vi "Project XML Editor.vi"() -> ()   [LabVIEW 2019]
uses:
  Project XML Editor/TypeDefs/Dependency Parameters.ctl
  Project XML Editor/Project XML Editor.lvclass
panel:
  out "Array":T1[](array[typedef])
  out "error out":errorcluster
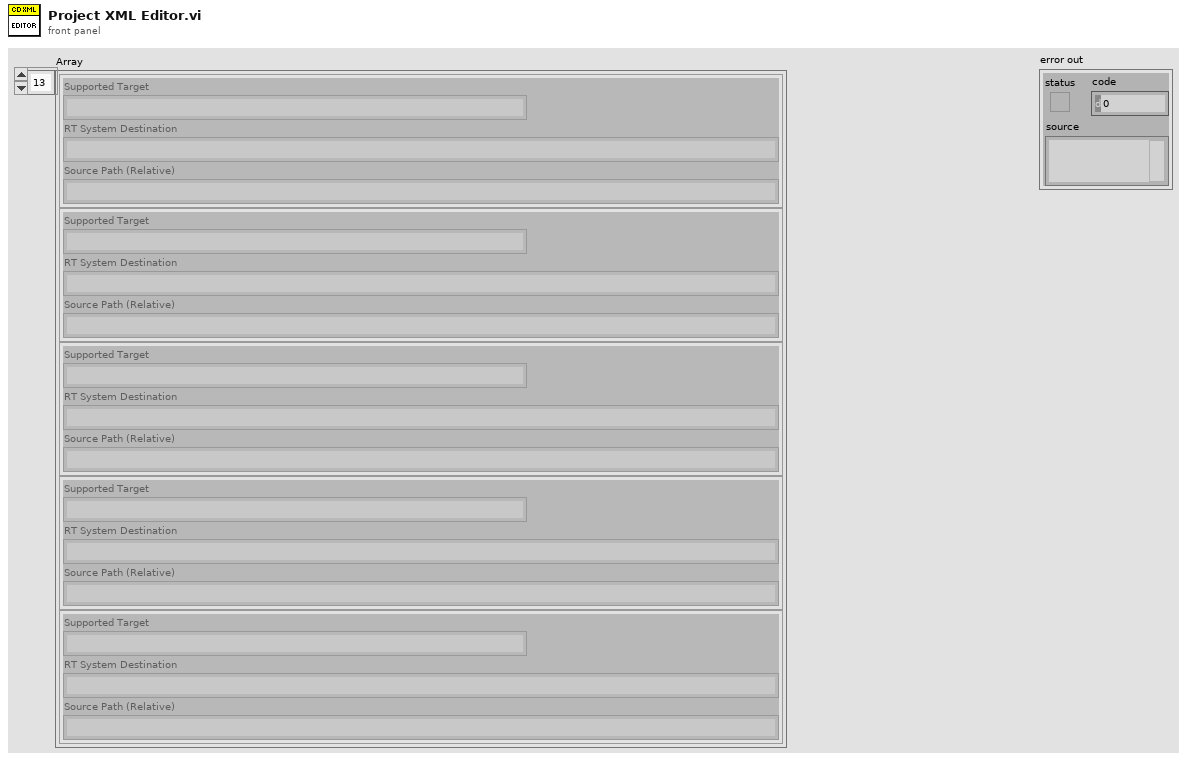
[diagram p1: front panel]
types:
  T1 = typedef "Project XML Editor.lvclass/Dependency Parameters.ctl" = cluster{"Supported Target":string, "RT System Destination":string, "Source Path (Relative)":string}
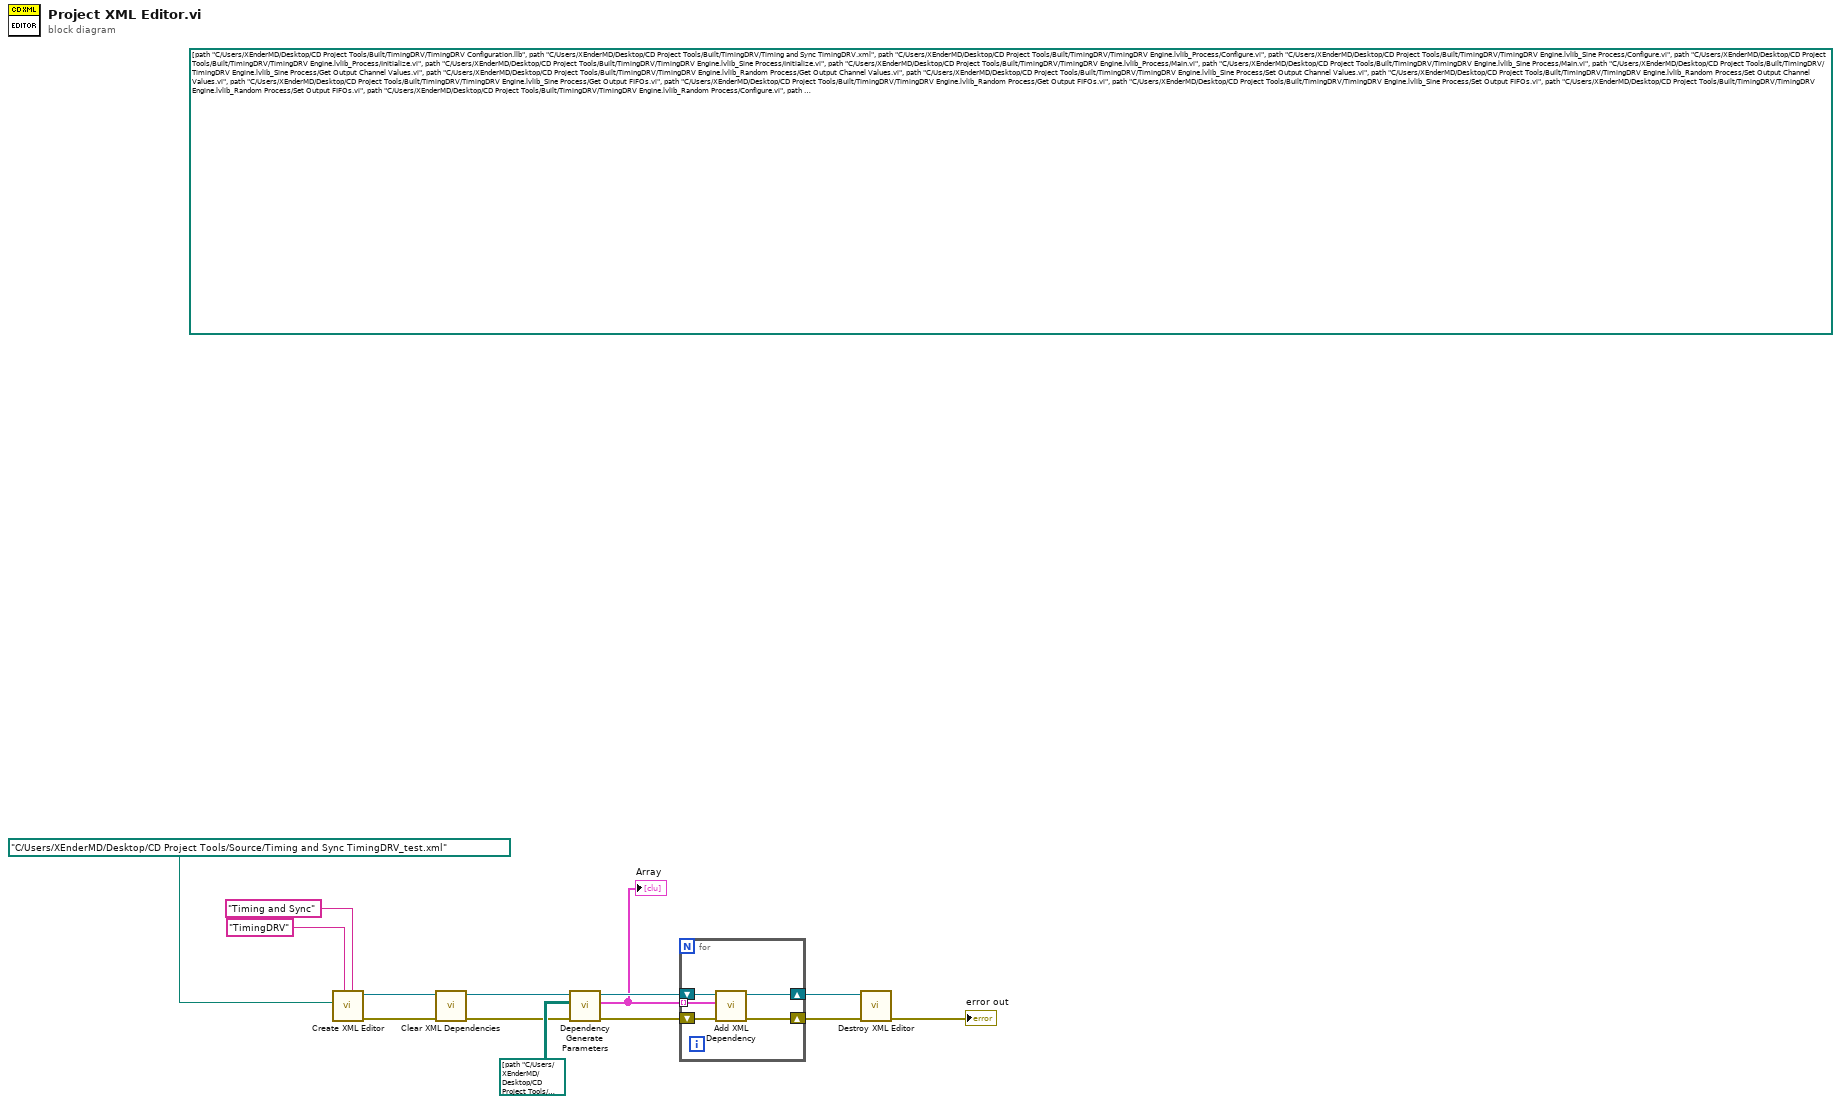
[diagram p0: block diagram]
diagram:
  (unwired) path[][] [[path "C:/Users/XEnderMD/Desktop/CD Project Tools/Built/TimingDRV/TimingDRV Configuration.llb", path "C:/Users/XEnderMD/Desktop/CD Project Tools/Built/TimingDRV/Timing and Sync TimingDRV.xml", path "C:/Users/XEnderMD/Desktop/CD Project Tools/Built/TimingDRV/TimingDRV Engine.lvlib_Process/Configure.vi", path "C:/Users/XEnderMD/Desktop/CD Project Tools/Built/TimingDRV/TimingDRV Engine.lvlib_Sine Process/Configure.vi", path "C:/Users/XEnderMD/Desktop/CD Project Tools/Built/TimingDRV/TimingDRV Engine.lvlib_Process/Initialize.vi", path "C:/Users/XEnderMD/Desktop/CD Project Tools/Built/TimingDRV/TimingDRV Engine.lvlib_Sine Process/Initialize.vi", path "C:/Users/XEnderMD/Desktop/CD Project Tools/Built/TimingDRV/TimingDRV Engine.lvlib_Process/Main.vi", path "C:/Users/XEnderMD/Desktop/CD Project Tools/Built/TimingDRV/TimingDRV Engine.lvlib_Sine Process/Main.vi", path "C:/Users/XEnderMD/Desktop/CD Project Tools/Built/TimingDRV/TimingDRV Engine.lvlib_Sine Process/Get Output Channel Values.vi", path "C:/Users/XEnderMD/Desktop/CD Project Tools/Built/TimingDRV/TimingDRV Engine.lvlib_Random Process/Get Output Channel Values.vi", path "C:/Users/XEnderMD/Desktop/CD Project Tools/Built/TimingDRV/TimingDRV Engine.lvlib_Sine Process/Set Output Channel Values.vi", path "C:/Users/XEnderMD/Desktop/CD Project Tools/Built/TimingDRV/TimingDRV Engine.lvlib_Random Process/Set Output Channel Values.vi", path "C:/Users/XEnderMD/Desktop/CD Project Tools/Built/TimingDRV/TimingDRV Engine.lvlib_Sine Process/Get Output FIFOs.vi", path "C:/Users/XEnderMD/Desktop/CD Project Tools/Built/TimingDRV/TimingDRV Engine.lvlib_Random Process/Get Output FIFOs.vi", path "C:/Users/XEnderMD/Desktop/CD Project Tools/Built/TimingDRV/TimingDRV Engine.lvlib_Sine Process/Set Output FIFOs.vi", path "C:/Users/XEnderMD/Desktop/CD Project Tools/Built/TimingDRV/TimingDRV Engine.lvlib_Random Process/Set Output FIFOs.vi", path "C:/Users/XEnderMD/Desktop/CD Project Tools/Built/TimingDRV/TimingDRV Engine.lvlib_Random Process/Configure.vi", path "C:/Users/XEnderMD/Desktop/CD Project Tools/Built/TimingDRV/TimingDRV Engine.lvlib_Random Process/Initialize.vi", path "C:/Users/XEnderMD/Desktop/CD Project Tools/Built/TimingDRV/TimingDRV Engine.lvlib_Sine Process/Initialize Output Channel Values.vi", path "C:/Users/XEnderMD/Desktop/CD Project Tools/Built/TimingDRV/TimingDRV Engine.lvlib_Random Process/Initialize Output Channel Values.vi", path "C:/Users/XEnderMD/Desktop/CD Project Tools/Built/TimingDRV/TimingDRV Engine.lvlib_Random Process/Main.vi", path "C:/Users/XEnderMD/Desktop/CD Project Tools/Built/TimingDRV/TimingDRV Engine.lvlib_Sine Process/Update Channel Value.vi", path "C:/Users/XEnderMD/Desktop/CD Project Tools/Built/TimingDRV/TimingDRV Engine.lvlib_Random Process/Update Channel Value.vi", path "", path "", path "", path "", path "", path "", path "", path "", path "", path "", path "", path "", path "", path "", path "", path "", path ""], [path "C:/Users/XEnderMD/Desktop/CD Project Tools/Built/TimingDRV/Windows/TimingDRV Engine Windows.llb", path "C:/Users/XEnderMD/Desktop/CD Project Tools/Built/TimingDRV/Windows/TimingDRV Engine.lvlib_Assembler/Main.vi", path "C:/Users/XEnderMD/Desktop/CD Project Tools/Built/TimingDRV/Windows/TimingDRV Engine.lvlib_Input Process/Main.vi", path "C:/Users/XEnderMD/Desktop/CD Project Tools/Built/TimingDRV/Windows/TimingDRV Engine.lvlib_Output Process/Initialize Output Channel Values.vi", path "C:/Users/XEnderMD/Desktop/CD Project Tools/Built/TimingDRV/Windows/TimingDRV Engine.lvlib_Sine Process/Initialize Output Channel Values.vi", path "C:/Users/XEnderMD/Desktop/CD Project Tools/Built/TimingDRV/Windows/TimingDRV Engine.lvlib_Output Process/Update Channel Value.vi", path "C:/Users/XEnderMD/Desktop/CD Project Tools/Built/TimingDRV/Windows/TimingDRV Engine.lvlib_Sine Process/Update Channel Value.vi", path "C:/Users/XEnderMD/Desktop/CD Project Tools/Built/TimingDRV/Windows/TimingDRV Engine.lvlib_Random Process/Initialize Output Channel Values.vi", path "C:/Users/XEnderMD/Desktop/CD Project Tools/Built/TimingDRV/Windows/TimingDRV Engine.lvlib_Random Process/Update Channel Value.vi", path "C:/Users/XEnderMD/Desktop/CD Project Tools/Built/TimingDRV/Windows/TimingDRV Engine.lvlib_Assembler/Configure.vi", path "C:/Users/XEnderMD/Desktop/CD Project Tools/Built/TimingDRV/Windows/TimingDRV Engine.lvlib_Output Process/Configure.vi", path "C:/Users/XEnderMD/Desktop/CD Project Tools/Built/TimingDRV/Windows/TimingDRV Engine.lvlib_Assembler/Initialize.vi", path "C:/Users/XEnderMD/Desktop/CD Project Tools/Built/TimingDRV/Windows/TimingDRV Engine.lvlib_Output Process/Initialize.vi", path "C:/Users/XEnderMD/Desktop/CD Project Tools/Built/TimingDRV/Windows/TimingDRV Engine.lvlib_Output Process/Main.vi", path "C:/Users/XEnderMD/Desktop/CD Project Tools/Built/TimingDRV/Windows/TimingDRV Engine.lvlib_Output Process/Get Output Channel Values.vi", path "C:/Users/XEnderMD/Desktop/CD Project Tools/Built/TimingDRV/Windows/TimingDRV Engine.lvlib_Sine Process/Get Output Channel Values.vi", path "C:/Users/XEnderMD/Desktop/CD Project Tools/Built/TimingDRV/Windows/TimingDRV Engine.lvlib_Output Process/Set Output Channel Values.vi", path "C:/Users/XEnderMD/Desktop/CD Project Tools/Built/TimingDRV/Windows/TimingDRV Engine.lvlib_Sine Process/Set Output Channel Values.vi", path "C:/Users/XEnderMD/Desktop/CD Project Tools/Built/TimingDRV/Windows/TimingDRV Engine.lvlib_Output Process/Get Output FIFOs.vi", path "C:/Users/XEnderMD/Desktop/CD Project Tools/Built/TimingDRV/Windows/TimingDRV Engine.lvlib_Sine Process/Get Output FIFOs.vi", path "C:/Users/XEnderMD/Desktop/CD Project Tools/Built/TimingDRV/Windows/TimingDRV Engine.lvlib_Output Process/Set Output FIFOs.vi", path "C:/Users/XEnderMD/Desktop/CD Project Tools/Built/TimingDRV/Windows/TimingDRV Engine.lvlib_Sine Process/Set Output FIFOs.vi", path "C:/Users/XEnderMD/Desktop/CD Project Tools/Built/TimingDRV/Windows/TimingDRV Engine.lvlib_Sine Process/Configure.vi", path "C:/Users/XEnderMD/Desktop/CD Project Tools/Built/TimingDRV/Windows/TimingDRV Engine.lvlib_Sine Process/Initialize.vi", path "C:/Users/XEnderMD/Desktop/CD Project Tools/Built/TimingDRV/Windows/TimingDRV Engine.lvlib_Sine Process/Main.vi", path "C:/Users/XEnderMD/Desktop/CD Project Tools/Built/TimingDRV/Windows/TimingDRV Engine.lvlib_Random Process/Get Output Channel Values.vi", path "C:/Users/XEnderMD/Desktop/CD Project Tools/Built/TimingDRV/Windows/TimingDRV Engine.lvlib_Random Process/Set Output Channel Values.vi", path "C:/Users/XEnderMD/Desktop/CD Project Tools/Built/TimingDRV/Windows/TimingDRV Engine.lvlib_Random Process/Get Output FIFOs.vi", path "C:/Users/XEnderMD/Desktop/CD Project Tools/Built/TimingDRV/Windows/TimingDRV Engine.lvlib_Random Process/Set Output FIFOs.vi", path "C:/Users/XEnderMD/Desktop/CD Project Tools/Built/TimingDRV/Windows/TimingDRV Engine.lvlib_Random Process/Configure.vi", path "C:/Users/XEnderMD/Desktop/CD Project Tools/Built/TimingDRV/Windows/TimingDRV Engine.lvlib_Random Process/Initialize.vi", path "C:/Users/XEnderMD/Desktop/CD Project Tools/Built/TimingDRV/Windows/TimingDRV Engine.lvlib_Random Process/Main.vi", path "C:/Users/XEnderMD/Desktop/CD Project Tools/Built/TimingDRV/Windows/TimingDRV Engine.lvlib_Process/Configure.vi", path "C:/Users/XEnderMD/Desktop/CD Project Tools/Built/TimingDRV/Windows/TimingDRV Engine.lvlib_Assembler/Launcher.vi", path "C:/Users/XEnderMD/Desktop/CD Project Tools/Built/TimingDRV/Windows/TimingDRV Engine.lvlib_Process/Launcher.vi", path "C:/Users/XEnderMD/Desktop/CD Project Tools/Built/TimingDRV/Windows/TimingDRV Engine.lvlib_Process/Initialize.vi", path "C:/Users/XEnderMD/Desktop/CD Project Tools/Built/TimingDRV/Windows/TimingDRV Engine.lvlib_Process/Main.vi", path "C:/Users/XEnderMD/Desktop/CD Project Tools/Built/TimingDRV/Windows/TimingDRV Engine.lvlib_Assembler/Shutdown.vi", path "C:/Users/XEnderMD/Desktop/CD Project Tools/Built/TimingDRV/Windows/TimingDRV Engine.lvlib_Process/Shutdown.vi", path ""], [path "C:/Users/XEnderMD/Desktop/CD Project Tools/Built/TimingDRV/Pharlap/TimingDRV Engine Pharlap.llb", path "C:/Users/XEnderMD/Desktop/CD Project Tools/Built/TimingDRV/Pharlap/TimingDRV Engine.lvlib_Assembler/Main.vi", path "C:/Users/XEnderMD/Desktop/CD Project Tools/Built/TimingDRV/Pharlap/TimingDRV Engine.lvlib_Input Process/Main.vi", path "C:/Users/XEnderMD/Desktop/CD Project Tools/Built/TimingDRV/Pharlap/TimingDRV Engine.lvlib_Output Process/Initialize Output Channel Values.vi", path "C:/Users/XEnderMD/Desktop/CD Project Tools/Built/TimingDRV/Pharlap/TimingDRV Engine.lvlib_Sine Process/Initialize Output Channel Values.vi", path "C:/Users/XEnderMD/Desktop/CD Project Tools/Built/TimingDRV/Pharlap/TimingDRV Engine.lvlib_Output Process/Update Channel Value.vi", path "C:/Users/XEnderMD/Desktop/CD Project Tools/Built/TimingDRV/Pharlap/TimingDRV Engine.lvlib_Sine Process/Update Channel Value.vi", path "C:/Users/XEnderMD/Desktop/CD Project Tools/Built/TimingDRV/Pharlap/TimingDRV Engine.lvlib_Random Process/Initialize Output Channel Values.vi", path "C:/Users/XEnderMD/Desktop/CD Project Tools/Built/TimingDRV/Pharlap/TimingDRV Engine.lvlib_Random Process/Update Channel Value.vi", path "C:/Users/XEnderMD/Desktop/CD Project Tools/Built/TimingDRV/Pharlap/TimingDRV Engine.lvlib_Assembler/Configure.vi", path "C:/Users/XEnderMD/Desktop/CD Project Tools/Built/TimingDRV/Pharlap/TimingDRV Engine.lvlib_Output Process/Configure.vi", path "C:/Users/XEnderMD/Desktop/CD Project Tools/Built/TimingDRV/Pharlap/TimingDRV Engine.lvlib_Assembler/Initialize.vi", path "C:/Users/XEnderMD/Desktop/CD Project Tools/Built/TimingDRV/Pharlap/TimingDRV Engine.lvlib_Output Process/Initialize.vi", path "C:/Users/XEnderMD/Desktop/CD Project Tools/Built/TimingDRV/Pharlap/TimingDRV Engine.lvlib_Output Process/Main.vi", path "C:/Users/XEnderMD/Desktop/CD Project Tools/Built/TimingDRV/Pharlap/TimingDRV Engine.lvlib_Output Process/Get Output Channel Values.vi", path "C:/Users/XEnderMD/Desktop/CD Project Tools/Built/TimingDRV/Pharlap/TimingDRV Engine.lvlib_Sine Process/Get Output Channel Values.vi", path "C:/Users/XEnderMD/Desktop/CD Project Tools/Built/TimingDRV/Pharlap/TimingDRV Engine.lvlib_Output Process/Set Output Channel Values.vi", path "C:/Users/XEnderMD/Desktop/CD Project Tools/Built/TimingDRV/Pharlap/TimingDRV Engine.lvlib_Sine Process/Set Output Channel Values.vi", path "C:/Users/XEnderMD/Desktop/CD Project Tools/Built/TimingDRV/Pharlap/TimingDRV Engine.lvlib_Output Process/Get Output FIFOs.vi", path "C:/Users/XEnderMD/Desktop/CD Project Tools/Built/TimingDRV/Pharlap/TimingDRV Engine.lvlib_Sine Process/Get Output FIFOs.vi", path "C:/Users/XEnderMD/Desktop/CD Project Tools/Built/TimingDRV/Pharlap/TimingDRV Engine.lvlib_Output Process/Set Output FIFOs.vi", path "C:/Users/XEnderMD/Desktop/CD Project Tools/Built/TimingDRV/Pharlap/TimingDRV Engine.lvlib_Sine Process/Set Output FIFOs.vi", path "C:/Users/XEnderMD/Desktop/CD Project Tools/Built/TimingDRV/Pharlap/TimingDRV Engine.lvlib_Sine Process/Configure.vi", path "C:/Users/XEnderMD/Desktop/CD Project Tools/Built/TimingDRV/Pharlap/TimingDRV Engine.lvlib_Sine Process/Initialize.vi", path "C:/Users/XEnderMD/Desktop/CD Project Tools/Built/TimingDRV/Pharlap/TimingDRV Engine.lvlib_Sine Process/Main.vi", path "C:/Users/XEnderMD/Desktop/CD Project Tools/Built/TimingDRV/Pharlap/TimingDRV Engine.lvlib_Random Process/Get Output Channel Values.vi", path "C:/Users/XEnderMD/Desktop/CD Project Tools/Built/TimingDRV/Pharlap/TimingDRV Engine.lvlib_Random Process/Set Output Channel Values.vi", path "C:/Users/XEnderMD/Desktop/CD Project Tools/Built/TimingDRV/Pharlap/TimingDRV Engine.lvlib_Random Process/Get Output FIFOs.vi", path "C:/Users/XEnderMD/Desktop/CD Project Tools/Built/TimingDRV/Pharlap/TimingDRV Engine.lvlib_Random Process/Set Output FIFOs.vi", path "C:/Users/XEnderMD/Desktop/CD Project Tools/Built/TimingDRV/Pharlap/TimingDRV Engine.lvlib_Random Process/Configure.vi", path "C:/Users/XEnderMD/Desktop/CD Project Tools/Built/TimingDRV/Pharlap/TimingDRV Engine.lvlib_Random Process/Initialize.vi", path "C:/Users/XEnderMD/Desktop/CD Project Tools/Built/TimingDRV/Pharlap/TimingDRV Engine.lvlib_Random Process/Main.vi", path "C:/Users/XEnderMD/Desktop/CD Project Tools/Built/TimingDRV/Pharlap/TimingDRV Engine.lvlib_Process/Configure.vi", path "C:/Users/XEnderMD/Desktop/CD Project Tools/Built/TimingDRV/Pharlap/TimingDRV Engine.lvlib_Assembler/Launcher.vi", path "C:/Users/XEnderMD/Desktop/CD Project Tools/Built/TimingDRV/Pharlap/TimingDRV Engine.lvlib_Process/Launcher.vi", path "C:/Users/XEnderMD/Desktop/CD Project Tools/Built/TimingDRV/Pharlap/TimingDRV Engine.lvlib_Process/Initialize.vi", path "C:/Users/XEnderMD/Desktop/CD Project Tools/Built/TimingDRV/Pharlap/TimingDRV Engine.lvlib_Process/Main.vi", path "C:/Users/XEnderMD/Desktop/CD Project Tools/Built/TimingDRV/Pharlap/TimingDRV Engine.lvlib_Assembler/Shutdown.vi", path "C:/Users/XEnderMD/Desktop/CD Project Tools/Built/TimingDRV/Pharlap/TimingDRV Engine.lvlib_Process/Shutdown.vi", path "C:/Users/XEnderMD/Desktop/CD Project Tools/Built/TimingDRV/Engine Release_depinstr.bin"], [path "C:/Users/XEnderMD/Desktop/CD Project Tools/Built/TimingDRV/VxWorks/TimingDRV Engine VxWorks.llb", path "C:/Users/XEnderMD/Desktop/CD Project Tools/Built/TimingDRV/VxWorks/TimingDRV Engine.lvlib_Assembler/Main.vi", path "C:/Users/XEnderMD/Desktop/CD Project Tools/Built/TimingDRV/VxWorks/TimingDRV Engine.lvlib_Input Process/Main.vi", path "C:/Users/XEnderMD/Desktop/CD Project Tools/Built/TimingDRV/VxWorks/TimingDRV Engine.lvlib_Output Process/Initialize Output Channel Values.vi", path "C:/Users/XEnderMD/Desktop/CD Project Tools/Built/TimingDRV/VxWorks/TimingDRV Engine.lvlib_Sine Process/Initialize Output Channel Values.vi", path "C:/Users/XEnderMD/Desktop/CD Project Tools/Built/TimingDRV/VxWorks/TimingDRV Engine.lvlib_Output Process/Update Channel Value.vi", path "C:/Users/XEnderMD/Desktop/CD Project Tools/Built/TimingDRV/VxWorks/TimingDRV Engine.lvlib_Sine Process/Update Channel Value.vi", path "C:/Users/XEnderMD/Desktop/CD Project Tools/Built/TimingDRV/VxWorks/TimingDRV Engine.lvlib_Random Process/Initialize Output Channel Values.vi", path "C:/Users/XEnderMD/Desktop/CD Project Tools/Built/TimingDRV/VxWorks/TimingDRV Engine.lvlib_Random Process/Update Channel Value.vi", path "C:/Users/XEnderMD/Desktop/CD Project Tools/Built/TimingDRV/VxWorks/TimingDRV Engine.lvlib_Assembler/Configure.vi", path "C:/Users/XEnderMD/Desktop/CD Project Tools/Built/TimingDRV/VxWorks/TimingDRV Engine.lvlib_Output Process/Configure.vi", path "C:/Users/XEnderMD/Desktop/CD Project Tools/Built/TimingDRV/VxWorks/TimingDRV Engine.lvlib_Assembler/Initialize.vi", path "C:/Users/XEnderMD/Desktop/CD Project Tools/Built/TimingDRV/VxWorks/TimingDRV Engine.lvlib_Output Process/Initialize.vi", path "C:/Users/XEnderMD/Desktop/CD Project Tools/Built/TimingDRV/VxWorks/TimingDRV Engine.lvlib_Output Process/Main.vi", path "C:/Users/XEnderMD/Desktop/CD Project Tools/Built/TimingDRV/VxWorks/TimingDRV Engine.lvlib_Output Process/Get Output Channel Values.vi", path "C:/Users/XEnderMD/Desktop/CD Project Tools/Built/TimingDRV/VxWorks/TimingDRV Engine.lvlib_Sine Process/Get Output Channel Values.vi", path "C:/Users/XEnderMD/Desktop/CD Project Tools/Built/TimingDRV/VxWorks/TimingDRV Engine.lvlib_Output Process/Set Output Channel Values.vi", path "C:/Users/XEnderMD/Desktop/CD Project Tools/Built/TimingDRV/VxWorks/TimingDRV Engine.lvlib_Sine Process/Set Output Channel Values.vi", path "C:/Users/XEnderMD/Desktop/CD Project Tools/Built/TimingDRV/VxWorks/TimingDRV Engine.lvlib_Output Process/Get Output FIFOs.vi", path "C:/Users/XEnderMD/Desktop/CD Project Tools/Built/TimingDRV/VxWorks/TimingDRV Engine.lvlib_Sine Process/Get Output FIFOs.vi", path "C:/Users/XEnderMD/Desktop/CD Project Tools/Built/TimingDRV/VxWorks/TimingDRV Engine.lvlib_Output Process/Set Output FIFOs.vi", path "C:/Users/XEnderMD/Desktop/CD Project Tools/Built/TimingDRV/VxWorks/TimingDRV Engine.lvlib_Sine Process/Set Output FIFOs.vi", path "C:/Users/XEnderMD/Desktop/CD Project Tools/Built/TimingDRV/VxWorks/TimingDRV Engine.lvlib_Sine Process/Configure.vi", path "C:/Users/XEnderMD/Desktop/CD Project Tools/Built/TimingDRV/VxWorks/TimingDRV Engine.lvlib_Sine Process/Initialize.vi", path "C:/Users/XEnderMD/Desktop/CD Project Tools/Built/TimingDRV/VxWorks/TimingDRV Engine.lvlib_Sine Process/Main.vi", path "C:/Users/XEnderMD/Desktop/CD Project Tools/Built/TimingDRV/VxWorks/TimingDRV Engine.lvlib_Random Process/Get Output Channel Values.vi", path "C:/Users/XEnderMD/Desktop/CD Project Tools/Built/TimingDRV/VxWorks/TimingDRV Engine.lvlib_Random Process/Set Output Channel Values.vi", path "C:/Users/XEnderMD/Desktop/CD Project Tools/Built/TimingDRV/VxWorks/TimingDRV Engine.lvlib_Random Process/Get Output FIFOs.vi", path "C:/Users/XEnderMD/Desktop/CD Project Tools/Built/TimingDRV/VxWorks/TimingDRV Engine.lvlib_Random Process/Set Output FIFOs.vi", path "C:/Users/XEnderMD/Desktop/CD Project Tools/Built/TimingDRV/VxWorks/TimingDRV Engine.lvlib_Random Process/Configure.vi", path "C:/Users/XEnderMD/Desktop/CD Project Tools/Built/TimingDRV/VxWorks/TimingDRV Engine.lvlib_Random Process/Initialize.vi", path "C:/Users/XEnderMD/Desktop/CD Project Tools/Built/TimingDRV/VxWorks/TimingDRV Engine.lvlib_Random Process/Main.vi", path "C:/Users/XEnderMD/Desktop/CD Project Tools/Built/TimingDRV/VxWorks/TimingDRV Engine.lvlib_Process/Configure.vi", path "C:/Users/XEnderMD/Desktop/CD Project Tools/Built/TimingDRV/VxWorks/TimingDRV Engine.lvlib_Assembler/Launcher.vi", path "C:/Users/XEnderMD/Desktop/CD Project Tools/Built/TimingDRV/VxWorks/TimingDRV Engine.lvlib_Process/Launcher.vi", path "C:/Users/XEnderMD/Desktop/CD Project Tools/Built/TimingDRV/VxWorks/TimingDRV Engine.lvlib_Process/Initialize.vi", path "C:/Users/XEnderMD/Desktop/CD Project Tools/Built/TimingDRV/VxWorks/TimingDRV Engine.lvlib_Process/Main.vi", path "C:/Users/XEnderMD/Desktop/CD Project Tools/Built/TimingDRV/VxWorks/TimingDRV Engine.lvlib_Assembler/Shutdown.vi", path "C:/Users/XEnderMD/Desktop/CD Project Tools/Built/TimingDRV/VxWorks/TimingDRV Engine.lvlib_Process/Shutdown.vi", path "C:/Users/XEnderMD/Desktop/CD Project Tools/Built/TimingDRV/Engine Release_depinstr.bin"], [path "C:/Users/XEnderMD/Desktop/CD Project Tools/Built/TimingDRV/Linux_32_ARM/TimingDRV Engine LinuxARM.llb", path "C:/Users/XEnderMD/Desktop/CD Project Tools/Built/TimingDRV/Linux_32_ARM/TimingDRV Engine.lvlib_Assembler/Main.vi", path "C:/Users/XEnderMD/Desktop/CD Project Tools/Built/TimingDRV/Linux_32_ARM/TimingDRV Engine.lvlib_Input Process/Main.vi", path "C:/Users/XEnderMD/Desktop/CD Project Tools/Built/TimingDRV/Linux_32_ARM/TimingDRV Engine.lvlib_Output Process/Initialize Output Channel Values.vi", path "C:/Users/XEnderMD/Desktop/CD Project Tools/Built/TimingDRV/Linux_32_ARM/TimingDRV Engine.lvlib_Sine Process/Initialize Output Channel Values.vi", path "C:/Users/XEnderMD/Desktop/CD Project Tools/Built/TimingDRV/Linux_32_ARM/TimingDRV Engine.lvlib_Output Process/Update Channel Value.vi", path "C:/Users/XEnderMD/Desktop/CD Project Tools/Built/TimingDRV/Linux_32_ARM/TimingDRV Engine.lvlib_Sine Process/Update Channel Value.vi", path "C:/Users/XEnderMD/Desktop/CD Project Tools/Built/TimingDRV/Linux_32_ARM/TimingDRV Engine.lvlib_Random Process/Initialize Output Channel Values.vi", path "C:/Users/XEnderMD/Desktop/CD Project Tools/Built/TimingDRV/Linux_32_ARM/TimingDRV Engine.lvlib_Random Process/Update Channel Value.vi", path "C:/Users/XEnderMD/Desktop/CD Project Tools/Built/TimingDRV/Linux_32_ARM/TimingDRV Engine.lvlib_Assembler/Configure.vi", path "C:/Users/XEnderMD/Desktop/CD Project Tools/Built/TimingDRV/Linux_32_ARM/TimingDRV Engine.lvlib_Output Process/Configure.vi", path "C:/Users/XEnderMD/Desktop/CD Project Tools/Built/TimingDRV/Linux_32_ARM/TimingDRV Engine.lvlib_Assembler/Initialize.vi", path "C:/Users/XEnderMD/Desktop/CD Project Tools/Built/TimingDRV/Linux_32_ARM/TimingDRV Engine.lvlib_Output Process/Initialize.vi", path "C:/Users/XEnderMD/Desktop/CD Project Tools/Built/TimingDRV/Linux_32_ARM/TimingDRV Engine.lvlib_Output Process/Main.vi", path "C:/Users/XEnderMD/Desktop/CD Project Tools/Built/TimingDRV/Linux_32_ARM/TimingDRV Engine.lvlib_Output Process/Get Output Channel Values.vi", path "C:/Users/XEnderMD/Desktop/CD Project Tools/Built/TimingDRV/Linux_32_ARM/TimingDRV Engine.lvlib_Sine Process/Get Output Channel Values.vi", path "C:/Users/XEnderMD/Desktop/CD Project Tools/Built/TimingDRV/Linux_32_ARM/TimingDRV Engine.lvlib_Output Process/Set Output Channel Values.vi", path "C:/Users/XEnderMD/Desktop/CD Project Tools/Built/TimingDRV/Linux_32_ARM/TimingDRV Engine.lvlib_Sine Process/Set Output Channel Values.vi", path "C:/Users/XEnderMD/Desktop/CD Project Tools/Built/TimingDRV/Linux_32_ARM/TimingDRV Engine.lvlib_Output Process/Get Output FIFOs.vi", path "C:/Users/XEnderMD/Desktop/CD Project Tools/Built/TimingDRV/Linux_32_ARM/TimingDRV Engine.lvlib_Sine Process/Get Output FIFOs.vi", path "C:/Users/XEnderMD/Desktop/CD Project Tools/Built/TimingDRV/Linux_32_ARM/TimingDRV Engine.lvlib_Output Process/Set Output FIFOs.vi", path "C:/Users/XEnderMD/Desktop/CD Project Tools/Built/TimingDRV/Linux_32_ARM/TimingDRV Engine.lvlib_Sine Process/Set Output FIFOs.vi", path "C:/Users/XEnderMD/Desktop/CD Project Tools/Built/TimingDRV/Linux_32_ARM/TimingDRV Engine.lvlib_Sine Process/Configure.vi", path "C:/Users/XEnderMD/Desktop/CD Project Tools/Built/TimingDRV/Linux_32_ARM/TimingDRV Engine.lvlib_Sine Process/Initialize.vi", path "C:/Users/XEnderMD/Desktop/CD Project Tools/Built/TimingDRV/Linux_32_ARM/TimingDRV Engine.lvlib_Sine Process/Main.vi", path "C:/Users/XEnderMD/Desktop/CD Project Tools/Built/TimingDRV/Linux_32_ARM/TimingDRV Engine.lvlib_Random Process/Get Output Channel Values.vi", path "C:/Users/XEnderMD/Desktop/CD Project Tools/Built/TimingDRV/Linux_32_ARM/TimingDRV Engine.lvlib_Random Process/Set Output Channel Values.vi", path "C:/Users/XEnderMD/Desktop/CD Project Tools/Built/TimingDRV/Linux_32_ARM/TimingDRV Engine.lvlib_Random Process/Get Output FIFOs.vi", path "C:/Users/XEnderMD/Desktop/CD Project Tools/Built/TimingDRV/Linux_32_ARM/TimingDRV Engine.lvlib_Random Process/Set Output FIFOs.vi", path "C:/Users/XEnderMD/Desktop/CD Project Tools/Built/TimingDRV/Linux_32_ARM/TimingDRV Engine.lvlib_Random Process/Configure.vi", path "C:/Users/XEnderMD/Desktop/CD Project Tools/Built/TimingDRV/Linux_32_ARM/TimingDRV Engine.lvlib_Random Process/Initialize.vi", path "C:/Users/XEnderMD/Desktop/CD Project Tools/Built/TimingDRV/Linux_32_ARM/TimingDRV Engine.lvlib_Random Process/Main.vi", path "C:/Users/XEnderMD/Desktop/CD Project Tools/Built/TimingDRV/Linux_32_ARM/TimingDRV Engine.lvlib_Process/Configure.vi", path "C:/Users/XEnderMD/Desktop/CD Project Tools/Built/TimingDRV/Linux_32_ARM/TimingDRV Engine.lvlib_Assembler/Launcher.vi", path "C:/Users/XEnderMD/Desktop/CD Project Tools/Built/TimingDRV/Linux_32_ARM/TimingDRV Engine.lvlib_Process/Launcher.vi", path "C:/Users/XEnderMD/Desktop/CD Project Tools/Built/TimingDRV/Linux_32_ARM/TimingDRV Engine.lvlib_Process/Initialize.vi", path "C:/Users/XEnderMD/Desktop/CD Project Tools/Built/TimingDRV/Linux_32_ARM/TimingDRV Engine.lvlib_Process/Main.vi", path "C:/Users/XEnderMD/Desktop/CD Project Tools/Built/TimingDRV/Linux_32_ARM/TimingDRV Engine.lvlib_Assembler/Shutdown.vi", path "C:/Users/XEnderMD/Desktop/CD Project Tools/Built/TimingDRV/Linux_32_ARM/TimingDRV Engine.lvlib_Process/Shutdown.vi", path "C:/Users/XEnderMD/Desktop/CD Project Tools/Built/TimingDRV/Engine Release_depinstr.bin"], [path "C:/Users/XEnderMD/Desktop/CD Project Tools/Built/TimingDRV/Linux_x64/TimingDRV Engine Linux64.llb", path "C:/Users/XEnderMD/Desktop/CD Project Tools/Built/TimingDRV/Linux_x64/TimingDRV Engine.lvlib_Assembler/Main.vi", path "C:/Users/XEnderMD/Desktop/CD Project Tools/Built/TimingDRV/Linux_x64/TimingDRV Engine.lvlib_Input Process/Main.vi", path "C:/Users/XEnderMD/Desktop/CD Project Tools/Built/TimingDRV/Linux_x64/TimingDRV Engine.lvlib_Output Process/Initialize Output Channel Values.vi", path "C:/Users/XEnderMD/Desktop/CD Project Tools/Built/TimingDRV/Linux_x64/TimingDRV Engine.lvlib_Sine Process/Initialize Output Channel Values.vi", path "C:/Users/XEnderMD/Desktop/CD Project Tools/Built/TimingDRV/Linux_x64/TimingDRV Engine.lvlib_Output Process/Update Channel Value.vi", path "C:/Users/XEnderMD/Desktop/CD Project Tools/Built/TimingDRV/Linux_x64/TimingDRV Engine.lvlib_Sine Process/Update Channel Value.vi", path "C:/Users/XEnderMD/Desktop/CD Project Tools/Built/TimingDRV/Linux_x64/TimingDRV Engine.lvlib_Random Process/Initialize Output Channel Values.vi", path "C:/Users/XEnderMD/Desktop/CD Project Tools/Built/TimingDRV/Linux_x64/TimingDRV Engine.lvlib_Random Process/Update Channel Value.vi", path "C:/Users/XEnderMD/Desktop/CD Project Tools/Built/TimingDRV/Linux_x64/TimingDRV Engine.lvlib_Assembler/Configure.vi", path "C:/Users/XEnderMD/Desktop/CD Project Tools/Built/TimingDRV/Linux_x64/TimingDRV Engine.lvlib_Output Process/Configure.vi", path "C:/Users/XEnderMD/Desktop/CD Project Tools/Built/TimingDRV/Linux_x64/TimingDRV Engine.lvlib_Assembler/Initialize.vi", path "C:/Users/XEnderMD/Desktop/CD Project Tools/Built/TimingDRV/Linux_x64/TimingDRV Engine.lvlib_Output Process/Initialize.vi", path "C:/Users/XEnderMD/Desktop/CD Project Tools/Built/TimingDRV/Linux_x64/TimingDRV Engine.lvlib_Output Process/Main.vi", path "C:/Users/XEnderMD/Desktop/CD Project Tools/Built/TimingDRV/Linux_x64/TimingDRV Engine.lvlib_Output Process/Get Output Channel Values.vi", path "C:/Users/XEnderMD/Desktop/CD Project Tools/Built/TimingDRV/Linux_x64/TimingDRV Engine.lvlib_Sine Process/Get Output Channel Values.vi", path "C:/Users/XEnderMD/Desktop/CD Project Tools/Built/TimingDRV/Linux_x64/TimingDRV Engine.lvlib_Output Process/Set Output Channel Values.vi", path "C:/Users/XEnderMD/Desktop/CD Project Tools/Built/TimingDRV/Linux_x64/TimingDRV Engine.lvlib_Sine Process/Set Output Channel Values.vi", path "C:/Users/XEnderMD/Desktop/CD Project Tools/Built/TimingDRV/Linux_x64/TimingDRV Engine.lvlib_Output Process/Get Output FIFOs.vi", path "C:/Users/XEnderMD/Desktop/CD Project Tools/Built/TimingDRV/Linux_x64/TimingDRV Engine.lvlib_Sine Process/Get Output FIFOs.vi", path "C:/Users/XEnderMD/Desktop/CD Project Tools/Built/TimingDRV/Linux_x64/TimingDRV Engine.lvlib_Output Process/Set Output FIFOs.vi", path "C:/Users/XEnderMD/Desktop/CD Project Tools/Built/TimingDRV/Linux_x64/TimingDRV Engine.lvlib_Sine Process/Set Output FIFOs.vi", path "C:/Users/XEnderMD/Desktop/CD Project Tools/Built/TimingDRV/Linux_x64/TimingDRV Engine.lvlib_Sine Process/Configure.vi", path "C:/Users/XEnderMD/Desktop/CD Project Tools/Built/TimingDRV/Linux_x64/TimingDRV Engine.lvlib_Sine Process/Initialize.vi", path "C:/Users/XEnderMD/Desktop/CD Project Tools/Built/TimingDRV/Linux_x64/TimingDRV Engine.lvlib_Sine Process/Main.vi", path "C:/Users/XEnderMD/Desktop/CD Project Tools/Built/TimingDRV/Linux_x64/TimingDRV Engine.lvlib_Random Process/Get Output Channel Values.vi", path "C:/Users/XEnderMD/Desktop/CD Project Tools/Built/TimingDRV/Linux_x64/TimingDRV Engine.lvlib_Random Process/Set Output Channel Values.vi", path "C:/Users/XEnderMD/Desktop/CD Project Tools/Built/TimingDRV/Linux_x64/TimingDRV Engine.lvlib_Random Process/Get Output FIFOs.vi", path "C:/Users/XEnderMD/Desktop/CD Project Tools/Built/TimingDRV/Linux_x64/TimingDRV Engine.lvlib_Random Process/Set Output FIFOs.vi", path "C:/Users/XEnderMD/Desktop/CD Project Tools/Built/TimingDRV/Linux_x64/TimingDRV Engine.lvlib_Random Process/Configure.vi", path "C:/Users/XEnderMD/Desktop/CD Project Tools/Built/TimingDRV/Linux_x64/TimingDRV Engine.lvlib_Random Process/Initialize.vi", path "C:/Users/XEnderMD/Desktop/CD Project Tools/Built/TimingDRV/Linux_x64/TimingDRV Engine.lvlib_Random Process/Main.vi", path "C:/Users/XEnderMD/Desktop/CD Project Tools/Built/TimingDRV/Linux_x64/TimingDRV Engine.lvlib_Process/Configure.vi", path "C:/Users/XEnderMD/Desktop/CD Project Tools/Built/TimingDRV/Linux_x64/TimingDRV Engine.lvlib_Assembler/Launcher.vi", path "C:/Users/XEnderMD/Desktop/CD Project Tools/Built/TimingDRV/Linux_x64/TimingDRV Engine.lvlib_Process/Launcher.vi", path "C:/Users/XEnderMD/Desktop/CD Project Tools/Built/TimingDRV/Linux_x64/TimingDRV Engine.lvlib_Process/Initialize.vi", path "C:/Users/XEnderMD/Desktop/CD Project Tools/Built/TimingDRV/Linux_x64/TimingDRV Engine.lvlib_Process/Main.vi", path "C:/Users/XEnderMD/Desktop/CD Project Tools/Built/TimingDRV/Linux_x64/TimingDRV Engine.lvlib_Assembler/Shutdown.vi", path "C:/Users/XEnderMD/Desktop/CD Project Tools/Built/TimingDRV/Linux_x64/TimingDRV Engine.lvlib_Process/Shutdown.vi", path "C:/Users/XEnderMD/Desktop/CD Project Tools/Built/TimingDRV/Engine Release_depinstr.bin"]] ("Generated files 2")
  n1 = call "Create XML Editor.vi"("Common Doc Dir"="Timing and Sync", "CD Name"="TimingDRV", "XML Path"=path "C:/Users/XEnderMD/Desktop/CD Project Tools/Source/Timing and Sync TimingDRV_test.xml") -> ("error out"=w8:errorcluster, "Project XML Editor out"=w9:refnum<class "Project XML Editor.lvclass">)  [unwired: 7 in]
  n2 = call "Clear XML Dependencies.vi"("error in (no error)"=w8, "Project XML Editor in"=w9) -> ("error out"=w5:errorcluster, "Project XML Editor out"=w4:refnum<class "Project XML Editor.lvclass">)  [unwired: 8 in]
  n3 = call "Dependency Generate Parameters.vi"("error in (no error)"=w5, "Generated files in"=path[][] [[path "C:/Users/XEnderMD/Desktop/CD Project Tools/Built/TimingDRV/TimingDRV Configuration.llb", path "C:/Users/XEnderMD/Desktop/CD Project Tools/Built/TimingDRV/Timing and Sync TimingDRV.xml", path "C:/Users/XEnderMD/Desktop/CD Project Tools/Built/TimingDRV/TimingDRV Engine.lvlib_Process/Configure.vi", path "C:/Users/XEnderMD/Desktop/CD Project Tools/Built/TimingDRV/TimingDRV Engine.lvlib_Sine Process/Configure.vi", path "C:/Users/XEnderMD/Desktop/CD Project Tools/Built/TimingDRV/TimingDRV Engine.lvlib_Process/Initialize.vi", path "C:/Users/XEnderMD/Desktop/CD Project Tools/Built/TimingDRV/TimingDRV Engine.lvlib_Sine Process/Initialize.vi", path "C:/Users/XEnderMD/Desktop/CD Project Tools/Built/TimingDRV/TimingDRV Engine.lvlib_Process/Main.vi", path "C:/Users/XEnderMD/Desktop/CD Project Tools/Built/TimingDRV/TimingDRV Engine.lvlib_Sine Process/Main.vi", path "C:/Users/XEnderMD/Desktop/CD Project Tools/Built/TimingDRV/TimingDRV Engine.lvlib_Sine Process/Get Output Channel Values.vi", path "C:/Users/XEnderMD/Desktop/CD Project Tools/Built/TimingDRV/TimingDRV Engine.lvlib_Random Process/Get Output Channel Values.vi", path "C:/Users/XEnderMD/Desktop/CD Project Tools/Built/TimingDRV/TimingDRV Engine.lvlib_Sine Process/Set Output Channel Values.vi", path "C:/Users/XEnderMD/Desktop/CD Project Tools/Built/TimingDRV/TimingDRV Engine.lvlib_Random Process/Set Output Channel Values.vi", path "C:/Users/XEnderMD/Desktop/CD Project Tools/Built/TimingDRV/TimingDRV Engine.lvlib_Sine Process/Get Output FIFOs.vi", path "C:/Users/XEnderMD/Desktop/CD Project Tools/Built/TimingDRV/TimingDRV Engine.lvlib_Random Process/Get Output FIFOs.vi", path "C:/Users/XEnderMD/Desktop/CD Project Tools/Built/TimingDRV/TimingDRV Engine.lvlib_Sine Process/Set Output FIFOs.vi", path "C:/Users/XEnderMD/Desktop/CD Project Tools/Built/TimingDRV/TimingDRV Engine.lvlib_Random Process/Set Output FIFOs.vi", path "C:/Users/XEnderMD/Desktop/CD Project Tools/Built/TimingDRV/TimingDRV Engine.lvlib_Random Process/Configure.vi", path "C:/Users/XEnderMD/Desktop/CD Project Tools/Built/TimingDRV/TimingDRV Engine.lvlib_Random Process/Initialize.vi", path "C:/Users/XEnderMD/Desktop/CD Project Tools/Built/TimingDRV/TimingDRV Engine.lvlib_Sine Process/Initialize Output Channel Values.vi", path "C:/Users/XEnderMD/Desktop/CD Project Tools/Built/TimingDRV/TimingDRV Engine.lvlib_Random Process/Initialize Output Channel Values.vi", path "C:/Users/XEnderMD/Desktop/CD Project Tools/Built/TimingDRV/TimingDRV Engine.lvlib_Random Process/Main.vi", path "C:/Users/XEnderMD/Desktop/CD Project Tools/Built/TimingDRV/TimingDRV Engine.lvlib_Sine Process/Update Channel Value.vi", path "C:/Users/XEnderMD/Desktop/CD Project Tools/Built/TimingDRV/TimingDRV Engine.lvlib_Random Process/Update Channel Value.vi", path "", path "", path "", path "", path "", path "", path "", path "", path "", path "", path "", path "", path "", path "", path "", path "", path ""], [path "C:/Users/XEnderMD/Desktop/CD Project Tools/Built/TimingDRV/Windows/TimingDRV Engine Windows.llb", path "C:/Users/XEnderMD/Desktop/CD Project Tools/Built/TimingDRV/Windows/TimingDRV Engine.lvlib_Assembler/Main.vi", path "C:/Users/XEnderMD/Desktop/CD Project Tools/Built/TimingDRV/Windows/TimingDRV Engine.lvlib_Input Process/Main.vi", path "C:/Users/XEnderMD/Desktop/CD Project Tools/Built/TimingDRV/Windows/TimingDRV Engine.lvlib_Output Process/Initialize Output Channel Values.vi", path "C:/Users/XEnderMD/Desktop/CD Project Tools/Built/TimingDRV/Windows/TimingDRV Engine.lvlib_Sine Process/Initialize Output Channel Values.vi", path "C:/Users/XEnderMD/Desktop/CD Project Tools/Built/TimingDRV/Windows/TimingDRV Engine.lvlib_Output Process/Update Channel Value.vi", path "C:/Users/XEnderMD/Desktop/CD Project Tools/Built/TimingDRV/Windows/TimingDRV Engine.lvlib_Sine Process/Update Channel Value.vi", path "C:/Users/XEnderMD/Desktop/CD Project Tools/Built/TimingDRV/Windows/TimingDRV Engine.lvlib_Random Process/Initialize Output Channel Values.vi", path "C:/Users/XEnderMD/Desktop/CD Project Tools/Built/TimingDRV/Windows/TimingDRV Engine.lvlib_Random Process/Update Channel Value.vi", path "C:/Users/XEnderMD/Desktop/CD Project Tools/Built/TimingDRV/Windows/TimingDRV Engine.lvlib_Assembler/Configure.vi", path "C:/Users/XEnderMD/Desktop/CD Project Tools/Built/TimingDRV/Windows/TimingDRV Engine.lvlib_Output Process/Configure.vi", path "C:/Users/XEnderMD/Desktop/CD Project Tools/Built/TimingDRV/Windows/TimingDRV Engine.lvlib_Assembler/Initialize.vi", path "C:/Users/XEnderMD/Desktop/CD Project Tools/Built/TimingDRV/Windows/TimingDRV Engine.lvlib_Output Process/Initialize.vi", path "C:/Users/XEnderMD/Desktop/CD Project Tools/Built/TimingDRV/Windows/TimingDRV Engine.lvlib_Output Process/Main.vi", path "C:/Users/XEnderMD/Desktop/CD Project Tools/Built/TimingDRV/Windows/TimingDRV Engine.lvlib_Output Process/Get Output Channel Values.vi", path "C:/Users/XEnderMD/Desktop/CD Project Tools/Built/TimingDRV/Windows/TimingDRV Engine.lvlib_Sine Process/Get Output Channel Values.vi", path "C:/Users/XEnderMD/Desktop/CD Project Tools/Built/TimingDRV/Windows/TimingDRV Engine.lvlib_Output Process/Set Output Channel Values.vi", path "C:/Users/XEnderMD/Desktop/CD Project Tools/Built/TimingDRV/Windows/TimingDRV Engine.lvlib_Sine Process/Set Output Channel Values.vi", path "C:/Users/XEnderMD/Desktop/CD Project Tools/Built/TimingDRV/Windows/TimingDRV Engine.lvlib_Output Process/Get Output FIFOs.vi", path "C:/Users/XEnderMD/Desktop/CD Project Tools/Built/TimingDRV/Windows/TimingDRV Engine.lvlib_Sine Process/Get Output FIFOs.vi", path "C:/Users/XEnderMD/Desktop/CD Project Tools/Built/TimingDRV/Windows/TimingDRV Engine.lvlib_Output Process/Set Output FIFOs.vi", path "C:/Users/XEnderMD/Desktop/CD Project Tools/Built/TimingDRV/Windows/TimingDRV Engine.lvlib_Sine Process/Set Output FIFOs.vi", path "C:/Users/XEnderMD/Desktop/CD Project Tools/Built/TimingDRV/Windows/TimingDRV Engine.lvlib_Sine Process/Configure.vi", path "C:/Users/XEnderMD/Desktop/CD Project Tools/Built/TimingDRV/Windows/TimingDRV Engine.lvlib_Sine Process/Initialize.vi", path "C:/Users/XEnderMD/Desktop/CD Project Tools/Built/TimingDRV/Windows/TimingDRV Engine.lvlib_Sine Process/Main.vi", path "C:/Users/XEnderMD/Desktop/CD Project Tools/Built/TimingDRV/Windows/TimingDRV Engine.lvlib_Random Process/Get Output Channel Values.vi", path "C:/Users/XEnderMD/Desktop/CD Project Tools/Built/TimingDRV/Windows/TimingDRV Engine.lvlib_Random Process/Set Output Channel Values.vi", path "C:/Users/XEnderMD/Desktop/CD Project Tools/Built/TimingDRV/Windows/TimingDRV Engine.lvlib_Random Process/Get Output FIFOs.vi", path "C:/Users/XEnderMD/Desktop/CD Project Tools/Built/TimingDRV/Windows/TimingDRV Engine.lvlib_Random Process/Set Output FIFOs.vi", path "C:/Users/XEnderMD/Desktop/CD Project Tools/Built/TimingDRV/Windows/TimingDRV Engine.lvlib_Random Process/Configure.vi", path "C:/Users/XEnderMD/Desktop/CD Project Tools/Built/TimingDRV/Windows/TimingDRV Engine.lvlib_Random Process/Initialize.vi", path "C:/Users/XEnderMD/Desktop/CD Project Tools/Built/TimingDRV/Windows/TimingDRV Engine.lvlib_Random Process/Main.vi", path "C:/Users/XEnderMD/Desktop/CD Project Tools/Built/TimingDRV/Windows/TimingDRV Engine.lvlib_Process/Configure.vi", path "C:/Users/XEnderMD/Desktop/CD Project Tools/Built/TimingDRV/Windows/TimingDRV Engine.lvlib_Assembler/Launcher.vi", path "C:/Users/XEnderMD/Desktop/CD Project Tools/Built/TimingDRV/Windows/TimingDRV Engine.lvlib_Process/Launcher.vi", path "C:/Users/XEnderMD/Desktop/CD Project Tools/Built/TimingDRV/Windows/TimingDRV Engine.lvlib_Process/Initialize.vi", path "C:/Users/XEnderMD/Desktop/CD Project Tools/Built/TimingDRV/Windows/TimingDRV Engine.lvlib_Process/Main.vi", path "C:/Users/XEnderMD/Desktop/CD Project Tools/Built/TimingDRV/Windows/TimingDRV Engine.lvlib_Assembler/Shutdown.vi", path "C:/Users/XEnderMD/Desktop/CD Project Tools/Built/TimingDRV/Windows/TimingDRV Engine.lvlib_Process/Shutdown.vi", path ""], [path "C:/Users/XEnderMD/Desktop/CD Project Tools/Built/TimingDRV/Pharlap/TimingDRV Engine Pharlap.llb", path "C:/Users/XEnderMD/Desktop/CD Project Tools/Built/TimingDRV/Pharlap/TimingDRV Engine.lvlib_Assembler/Main.vi", path "C:/Users/XEnderMD/Desktop/CD Project Tools/Built/TimingDRV/Pharlap/TimingDRV Engine.lvlib_Input Process/Main.vi", path "C:/Users/XEnderMD/Desktop/CD Project Tools/Built/TimingDRV/Pharlap/TimingDRV Engine.lvlib_Output Process/Initialize Output Channel Values.vi", path "C:/Users/XEnderMD/Desktop/CD Project Tools/Built/TimingDRV/Pharlap/TimingDRV Engine.lvlib_Sine Process/Initialize Output Channel Values.vi", path "C:/Users/XEnderMD/Desktop/CD Project Tools/Built/TimingDRV/Pharlap/TimingDRV Engine.lvlib_Output Process/Update Channel Value.vi", path "C:/Users/XEnderMD/Desktop/CD Project Tools/Built/TimingDRV/Pharlap/TimingDRV Engine.lvlib_Sine Process/Update Channel Value.vi", path "C:/Users/XEnderMD/Desktop/CD Project Tools/Built/TimingDRV/Pharlap/TimingDRV Engine.lvlib_Random Process/Initialize Output Channel Values.vi", path "C:/Users/XEnderMD/Desktop/CD Project Tools/Built/TimingDRV/Pharlap/TimingDRV Engine.lvlib_Random Process/Update Channel Value.vi", path "C:/Users/XEnderMD/Desktop/CD Project Tools/Built/TimingDRV/Pharlap/TimingDRV Engine.lvlib_Assembler/Configure.vi", path "C:/Users/XEnderMD/Desktop/CD Project Tools/Built/TimingDRV/Pharlap/TimingDRV Engine.lvlib_Output Process/Configure.vi", path "C:/Users/XEnderMD/Desktop/CD Project Tools/Built/TimingDRV/Pharlap/TimingDRV Engine.lvlib_Assembler/Initialize.vi", path "C:/Users/XEnderMD/Desktop/CD Project Tools/Built/TimingDRV/Pharlap/TimingDRV Engine.lvlib_Output Process/Initialize.vi", path "C:/Users/XEnderMD/Desktop/CD Project Tools/Built/TimingDRV/Pharlap/TimingDRV Engine.lvlib_Output Process/Main.vi", path "C:/Users/XEnderMD/Desktop/CD Project Tools/Built/TimingDRV/Pharlap/TimingDRV Engine.lvlib_Output Process/Get Output Channel Values.vi", path "C:/Users/XEnderMD/Desktop/CD Project Tools/Built/TimingDRV/Pharlap/TimingDRV Engine.lvlib_Sine Process/Get Output Channel Values.vi", path "C:/Users/XEnderMD/Desktop/CD Project Tools/Built/TimingDRV/Pharlap/TimingDRV Engine.lvlib_Output Process/Set Output Channel Values.vi", path "C:/Users/XEnderMD/Desktop/CD Project Tools/Built/TimingDRV/Pharlap/TimingDRV Engine.lvlib_Sine Process/Set Output Channel Values.vi", path "C:/Users/XEnderMD/Desktop/CD Project Tools/Built/TimingDRV/Pharlap/TimingDRV Engine.lvlib_Output Process/Get Output FIFOs.vi", path "C:/Users/XEnderMD/Desktop/CD Project Tools/Built/TimingDRV/Pharlap/TimingDRV Engine.lvlib_Sine Process/Get Output FIFOs.vi", path "C:/Users/XEnderMD/Desktop/CD Project Tools/Built/TimingDRV/Pharlap/TimingDRV Engine.lvlib_Output Process/Set Output FIFOs.vi", path "C:/Users/XEnderMD/Desktop/CD Project Tools/Built/TimingDRV/Pharlap/TimingDRV Engine.lvlib_Sine Process/Set Output FIFOs.vi", path "C:/Users/XEnderMD/Desktop/CD Project Tools/Built/TimingDRV/Pharlap/TimingDRV Engine.lvlib_Sine Process/Configure.vi", path "C:/Users/XEnderMD/Desktop/CD Project Tools/Built/TimingDRV/Pharlap/TimingDRV Engine.lvlib_Sine Process/Initialize.vi", path "C:/Users/XEnderMD/Desktop/CD Project Tools/Built/TimingDRV/Pharlap/TimingDRV Engine.lvlib_Sine Process/Main.vi", path "C:/Users/XEnderMD/Desktop/CD Project Tools/Built/TimingDRV/Pharlap/TimingDRV Engine.lvlib_Random Process/Get Output Channel Values.vi", path "C:/Users/XEnderMD/Desktop/CD Project Tools/Built/TimingDRV/Pharlap/TimingDRV Engine.lvlib_Random Process/Set Output Channel Values.vi", path "C:/Users/XEnderMD/Desktop/CD Project Tools/Built/TimingDRV/Pharlap/TimingDRV Engine.lvlib_Random Process/Get Output FIFOs.vi", path "C:/Users/XEnderMD/Desktop/CD Project Tools/Built/TimingDRV/Pharlap/TimingDRV Engine.lvlib_Random Process/Set Output FIFOs.vi", path "C:/Users/XEnderMD/Desktop/CD Project Tools/Built/TimingDRV/Pharlap/TimingDRV Engine.lvlib_Random Process/Configure.vi", path "C:/Users/XEnderMD/Desktop/CD Project Tools/Built/TimingDRV/Pharlap/TimingDRV Engine.lvlib_Random Process/Initialize.vi", path "C:/Users/XEnderMD/Desktop/CD Project Tools/Built/TimingDRV/Pharlap/TimingDRV Engine.lvlib_Random Process/Main.vi", path "C:/Users/XEnderMD/Desktop/CD Project Tools/Built/TimingDRV/Pharlap/TimingDRV Engine.lvlib_Process/Configure.vi", path "C:/Users/XEnderMD/Desktop/CD Project Tools/Built/TimingDRV/Pharlap/TimingDRV Engine.lvlib_Assembler/Launcher.vi", path "C:/Users/XEnderMD/Desktop/CD Project Tools/Built/TimingDRV/Pharlap/TimingDRV Engine.lvlib_Process/Launcher.vi", path "C:/Users/XEnderMD/Desktop/CD Project Tools/Built/TimingDRV/Pharlap/TimingDRV Engine.lvlib_Process/Initialize.vi", path "C:/Users/XEnderMD/Desktop/CD Project Tools/Built/TimingDRV/Pharlap/TimingDRV Engine.lvlib_Process/Main.vi", path "C:/Users/XEnderMD/Desktop/CD Project Tools/Built/TimingDRV/Pharlap/TimingDRV Engine.lvlib_Assembler/Shutdown.vi", path "C:/Users/XEnderMD/Desktop/CD Project Tools/Built/TimingDRV/Pharlap/TimingDRV Engine.lvlib_Process/Shutdown.vi", path "C:/Users/XEnderMD/Desktop/CD Project Tools/Built/TimingDRV/Engine Release_depinstr.bin"], [path "C:/Users/XEnderMD/Desktop/CD Project Tools/Built/TimingDRV/VxWorks/TimingDRV Engine VxWorks.llb", path "C:/Users/XEnderMD/Desktop/CD Project Tools/Built/TimingDRV/VxWorks/TimingDRV Engine.lvlib_Assembler/Main.vi", path "C:/Users/XEnderMD/Desktop/CD Project Tools/Built/TimingDRV/VxWorks/TimingDRV Engine.lvlib_Input Process/Main.vi", path "C:/Users/XEnderMD/Desktop/CD Project Tools/Built/TimingDRV/VxWorks/TimingDRV Engine.lvlib_Output Process/Initialize Output Channel Values.vi", path "C:/Users/XEnderMD/Desktop/CD Project Tools/Built/TimingDRV/VxWorks/TimingDRV Engine.lvlib_Sine Process/Initialize Output Channel Values.vi", path "C:/Users/XEnderMD/Desktop/CD Project Tools/Built/TimingDRV/VxWorks/TimingDRV Engine.lvlib_Output Process/Update Channel Value.vi", path "C:/Users/XEnderMD/Desktop/CD Project Tools/Built/TimingDRV/VxWorks/TimingDRV Engine.lvlib_Sine Process/Update Channel Value.vi", path "C:/Users/XEnderMD/Desktop/CD Project Tools/Built/TimingDRV/VxWorks/TimingDRV Engine.lvlib_Random Process/Initialize Output Channel Values.vi", path "C:/Users/XEnderMD/Desktop/CD Project Tools/Built/TimingDRV/VxWorks/TimingDRV Engine.lvlib_Random Process/Update Channel Value.vi", path "C:/Users/XEnderMD/Desktop/CD Project Tools/Built/TimingDRV/VxWorks/TimingDRV Engine.lvlib_Assembler/Configure.vi", path "C:/Users/XEnderMD/Desktop/CD Project Tools/Built/TimingDRV/VxWorks/TimingDRV Engine.lvlib_Output Process/Configure.vi", path "C:/Users/XEnderMD/Desktop/CD Project Tools/Built/TimingDRV/VxWorks/TimingDRV Engine.lvlib_Assembler/Initialize.vi", path "C:/Users/XEnderMD/Desktop/CD Project Tools/Built/TimingDRV/VxWorks/TimingDRV Engine.lvlib_Output Process/Initialize.vi", path "C:/Users/XEnderMD/Desktop/CD Project Tools/Built/TimingDRV/VxWorks/TimingDRV Engine.lvlib_Output Process/Main.vi", path "C:/Users/XEnderMD/Desktop/CD Project Tools/Built/TimingDRV/VxWorks/TimingDRV Engine.lvlib_Output Process/Get Output Channel Values.vi", path "C:/Users/XEnderMD/Desktop/CD Project Tools/Built/TimingDRV/VxWorks/TimingDRV Engine.lvlib_Sine Process/Get Output Channel Values.vi", path "C:/Users/XEnderMD/Desktop/CD Project Tools/Built/TimingDRV/VxWorks/TimingDRV Engine.lvlib_Output Process/Set Output Channel Values.vi", path "C:/Users/XEnderMD/Desktop/CD Project Tools/Built/TimingDRV/VxWorks/TimingDRV Engine.lvlib_Sine Process/Set Output Channel Values.vi", path "C:/Users/XEnderMD/Desktop/CD Project Tools/Built/TimingDRV/VxWorks/TimingDRV Engine.lvlib_Output Process/Get Output FIFOs.vi", path "C:/Users/XEnderMD/Desktop/CD Project Tools/Built/TimingDRV/VxWorks/TimingDRV Engine.lvlib_Sine Process/Get Output FIFOs.vi", path "C:/Users/XEnderMD/Desktop/CD Project Tools/Built/TimingDRV/VxWorks/TimingDRV Engine.lvlib_Output Process/Set Output FIFOs.vi", path "C:/Users/XEnderMD/Desktop/CD Project Tools/Built/TimingDRV/VxWorks/TimingDRV Engine.lvlib_Sine Process/Set Output FIFOs.vi", path "C:/Users/XEnderMD/Desktop/CD Project Tools/Built/TimingDRV/VxWorks/TimingDRV Engine.lvlib_Sine Process/Configure.vi", path "C:/Users/XEnderMD/Desktop/CD Project Tools/Built/TimingDRV/VxWorks/TimingDRV Engine.lvlib_Sine Process/Initialize.vi", path "C:/Users/XEnderMD/Desktop/CD Project Tools/Built/TimingDRV/VxWorks/TimingDRV Engine.lvlib_Sine Process/Main.vi", path "C:/Users/XEnderMD/Desktop/CD Project Tools/Built/TimingDRV/VxWorks/TimingDRV Engine.lvlib_Random Process/Get Output Channel Values.vi", path "C:/Users/XEnderMD/Desktop/CD Project Tools/Built/TimingDRV/VxWorks/TimingDRV Engine.lvlib_Random Process/Set Output Channel Values.vi", path "C:/Users/XEnderMD/Desktop/CD Project Tools/Built/TimingDRV/VxWorks/TimingDRV Engine.lvlib_Random Process/Get Output FIFOs.vi", path "C:/Users/XEnderMD/Desktop/CD Project Tools/Built/TimingDRV/VxWorks/TimingDRV Engine.lvlib_Random Process/Set Output FIFOs.vi", path "C:/Users/XEnderMD/Desktop/CD Project Tools/Built/TimingDRV/VxWorks/TimingDRV Engine.lvlib_Random Process/Configure.vi", path "C:/Users/XEnderMD/Desktop/CD Project Tools/Built/TimingDRV/VxWorks/TimingDRV Engine.lvlib_Random Process/Initialize.vi", path "C:/Users/XEnderMD/Desktop/CD Project Tools/Built/TimingDRV/VxWorks/TimingDRV Engine.lvlib_Random Process/Main.vi", path "C:/Users/XEnderMD/Desktop/CD Project Tools/Built/TimingDRV/VxWorks/TimingDRV Engine.lvlib_Process/Configure.vi", path "C:/Users/XEnderMD/Desktop/CD Project Tools/Built/TimingDRV/VxWorks/TimingDRV Engine.lvlib_Assembler/Launcher.vi", path "C:/Users/XEnderMD/Desktop/CD Project Tools/Built/TimingDRV/VxWorks/TimingDRV Engine.lvlib_Process/Launcher.vi", path "C:/Users/XEnderMD/Desktop/CD Project Tools/Built/TimingDRV/VxWorks/TimingDRV Engine.lvlib_Process/Initialize.vi", path "C:/Users/XEnderMD/Desktop/CD Project Tools/Built/TimingDRV/VxWorks/TimingDRV Engine.lvlib_Process/Main.vi", path "C:/Users/XEnderMD/Desktop/CD Project Tools/Built/TimingDRV/VxWorks/TimingDRV Engine.lvlib_Assembler/Shutdown.vi", path "C:/Users/XEnderMD/Desktop/CD Project Tools/Built/TimingDRV/VxWorks/TimingDRV Engine.lvlib_Process/Shutdown.vi", path "C:/Users/XEnderMD/Desktop/CD Project Tools/Built/TimingDRV/Engine Release_depinstr.bin"], [path "C:/Users/XEnderMD/Desktop/CD Project Tools/Built/TimingDRV/Linux_32_ARM/TimingDRV Engine LinuxARM.llb", path "C:/Users/XEnderMD/Desktop/CD Project Tools/Built/TimingDRV/Linux_32_ARM/TimingDRV Engine.lvlib_Assembler/Main.vi", path "C:/Users/XEnderMD/Desktop/CD Project Tools/Built/TimingDRV/Linux_32_ARM/TimingDRV Engine.lvlib_Input Process/Main.vi", path "C:/Users/XEnderMD/Desktop/CD Project Tools/Built/TimingDRV/Linux_32_ARM/TimingDRV Engine.lvlib_Output Process/Initialize Output Channel Values.vi", path "C:/Users/XEnderMD/Desktop/CD Project Tools/Built/TimingDRV/Linux_32_ARM/TimingDRV Engine.lvlib_Sine Process/Initialize Output Channel Values.vi", path "C:/Users/XEnderMD/Desktop/CD Project Tools/Built/TimingDRV/Linux_32_ARM/TimingDRV Engine.lvlib_Output Process/Update Channel Value.vi", path "C:/Users/XEnderMD/Desktop/CD Project Tools/Built/TimingDRV/Linux_32_ARM/TimingDRV Engine.lvlib_Sine Process/Update Channel Value.vi", path "C:/Users/XEnderMD/Desktop/CD Project Tools/Built/TimingDRV/Linux_32_ARM/TimingDRV Engine.lvlib_Random Process/Initialize Output Channel Values.vi", path "C:/Users/XEnderMD/Desktop/CD Project Tools/Built/TimingDRV/Linux_32_ARM/TimingDRV Engine.lvlib_Random Process/Update Channel Value.vi", path "C:/Users/XEnderMD/Desktop/CD Project Tools/Built/TimingDRV/Linux_32_ARM/TimingDRV Engine.lvlib_Assembler/Configure.vi", path "C:/Users/XEnderMD/Desktop/CD Project Tools/Built/TimingDRV/Linux_32_ARM/TimingDRV Engine.lvlib_Output Process/Configure.vi", path "C:/Users/XEnderMD/Desktop/CD Project Tools/Built/TimingDRV/Linux_32_ARM/TimingDRV Engine.lvlib_Assembler/Initialize.vi", path "C:/Users/XEnderMD/Desktop/CD Project Tools/Built/TimingDRV/Linux_32_ARM/TimingDRV Engine.lvlib_Output Process/Initialize.vi", path "C:/Users/XEnderMD/Desktop/CD Project Tools/Built/TimingDRV/Linux_32_ARM/TimingDRV Engine.lvlib_Output Process/Main.vi", path "C:/Users/XEnderMD/Desktop/CD Project Tools/Built/TimingDRV/Linux_32_ARM/TimingDRV Engine.lvlib_Output Process/Get Output Channel Values.vi", path "C:/Users/XEnderMD/Desktop/CD Project Tools/Built/TimingDRV/Linux_32_ARM/TimingDRV Engine.lvlib_Sine Process/Get Output Channel Values.vi", path "C:/Users/XEnderMD/Desktop/CD Project Tools/Built/TimingDRV/Linux_32_ARM/TimingDRV Engine.lvlib_Output Process/Set Output Channel Values.vi", path "C:/Users/XEnderMD/Desktop/CD Project Tools/Built/TimingDRV/Linux_32_ARM/TimingDRV Engine.lvlib_Sine Process/Set Output Channel Values.vi", path "C:/Users/XEnderMD/Desktop/CD Project Tools/Built/TimingDRV/Linux_32_ARM/TimingDRV Engine.lvlib_Output Process/Get Output FIFOs.vi", path "C:/Users/XEnderMD/Desktop/CD Project Tools/Built/TimingDRV/Linux_32_ARM/TimingDRV Engine.lvlib_Sine Process/Get Output FIFOs.vi", path "C:/Users/XEnderMD/Desktop/CD Project Tools/Built/TimingDRV/Linux_32_ARM/TimingDRV Engine.lvlib_Output Process/Set Output FIFOs.vi", path "C:/Users/XEnderMD/Desktop/CD Project Tools/Built/TimingDRV/Linux_32_ARM/TimingDRV Engine.lvlib_Sine Process/Set Output FIFOs.vi", path "C:/Users/XEnderMD/Desktop/CD Project Tools/Built/TimingDRV/Linux_32_ARM/TimingDRV Engine.lvlib_Sine Process/Configure.vi", path "C:/Users/XEnderMD/Desktop/CD Project Tools/Built/TimingDRV/Linux_32_ARM/TimingDRV Engine.lvlib_Sine Process/Initialize.vi", path "C:/Users/XEnderMD/Desktop/CD Project Tools/Built/TimingDRV/Linux_32_ARM/TimingDRV Engine.lvlib_Sine Process/Main.vi", path "C:/Users/XEnderMD/Desktop/CD Project Tools/Built/TimingDRV/Linux_32_ARM/TimingDRV Engine.lvlib_Random Process/Get Output Channel Values.vi", path "C:/Users/XEnderMD/Desktop/CD Project Tools/Built/TimingDRV/Linux_32_ARM/TimingDRV Engine.lvlib_Random Process/Set Output Channel Values.vi", path "C:/Users/XEnderMD/Desktop/CD Project Tools/Built/TimingDRV/Linux_32_ARM/TimingDRV Engine.lvlib_Random Process/Get Output FIFOs.vi", path "C:/Users/XEnderMD/Desktop/CD Project Tools/Built/TimingDRV/Linux_32_ARM/TimingDRV Engine.lvlib_Random Process/Set Output FIFOs.vi", path "C:/Users/XEnderMD/Desktop/CD Project Tools/Built/TimingDRV/Linux_32_ARM/TimingDRV Engine.lvlib_Random Process/Configure.vi", path "C:/Users/XEnderMD/Desktop/CD Project Tools/Built/TimingDRV/Linux_32_ARM/TimingDRV Engine.lvlib_Random Process/Initialize.vi", path "C:/Users/XEnderMD/Desktop/CD Project Tools/Built/TimingDRV/Linux_32_ARM/TimingDRV Engine.lvlib_Random Process/Main.vi", path "C:/Users/XEnderMD/Desktop/CD Project Tools/Built/TimingDRV/Linux_32_ARM/TimingDRV Engine.lvlib_Process/Configure.vi", path "C:/Users/XEnderMD/Desktop/CD Project Tools/Built/TimingDRV/Linux_32_ARM/TimingDRV Engine.lvlib_Assembler/Launcher.vi", path "C:/Users/XEnderMD/Desktop/CD Project Tools/Built/TimingDRV/Linux_32_ARM/TimingDRV Engine.lvlib_Process/Launcher.vi", path "C:/Users/XEnderMD/Desktop/CD Project Tools/Built/TimingDRV/Linux_32_ARM/TimingDRV Engine.lvlib_Process/Initialize.vi", path "C:/Users/XEnderMD/Desktop/CD Project Tools/Built/TimingDRV/Linux_32_ARM/TimingDRV Engine.lvlib_Process/Main.vi", path "C:/Users/XEnderMD/Desktop/CD Project Tools/Built/TimingDRV/Linux_32_ARM/TimingDRV Engine.lvlib_Assembler/Shutdown.vi", path "C:/Users/XEnderMD/Desktop/CD Project Tools/Built/TimingDRV/Linux_32_ARM/TimingDRV Engine.lvlib_Process/Shutdown.vi", path "C:/Users/XEnderMD/Desktop/CD Project Tools/Built/TimingDRV/Engine Release_depinstr.bin"], [path "C:/Users/XEnderMD/Desktop/CD Project Tools/Built/TimingDRV/Linux_x64/TimingDRV Engine Linux64.llb", path "C:/Users/XEnderMD/Desktop/CD Project Tools/Built/TimingDRV/Linux_x64/TimingDRV Engine.lvlib_Assembler/Main.vi", path "C:/Users/XEnderMD/Desktop/CD Project Tools/Built/TimingDRV/Linux_x64/TimingDRV Engine.lvlib_Input Process/Main.vi", path "C:/Users/XEnderMD/Desktop/CD Project Tools/Built/TimingDRV/Linux_x64/TimingDRV Engine.lvlib_Output Process/Initialize Output Channel Values.vi", path "C:/Users/XEnderMD/Desktop/CD Project Tools/Built/TimingDRV/Linux_x64/TimingDRV Engine.lvlib_Sine Process/Initialize Output Channel Values.vi", path "C:/Users/XEnderMD/Desktop/CD Project Tools/Built/TimingDRV/Linux_x64/TimingDRV Engine.lvlib_Output Process/Update Channel Value.vi", path "C:/Users/XEnderMD/Desktop/CD Project Tools/Built/TimingDRV/Linux_x64/TimingDRV Engine.lvlib_Sine Process/Update Channel Value.vi", path "C:/Users/XEnderMD/Desktop/CD Project Tools/Built/TimingDRV/Linux_x64/TimingDRV Engine.lvlib_Random Process/Initialize Output Channel Values.vi", path "C:/Users/XEnderMD/Desktop/CD Project Tools/Built/TimingDRV/Linux_x64/TimingDRV Engine.lvlib_Random Process/Update Channel Value.vi", path "C:/Users/XEnderMD/Desktop/CD Project Tools/Built/TimingDRV/Linux_x64/TimingDRV Engine.lvlib_Assembler/Configure.vi", path "C:/Users/XEnderMD/Desktop/CD Project Tools/Built/TimingDRV/Linux_x64/TimingDRV Engine.lvlib_Output Process/Configure.vi", path "C:/Users/XEnderMD/Desktop/CD Project Tools/Built/TimingDRV/Linux_x64/TimingDRV Engine.lvlib_Assembler/Initialize.vi", path "C:/Users/XEnderMD/Desktop/CD Project Tools/Built/TimingDRV/Linux_x64/TimingDRV Engine.lvlib_Output Process/Initialize.vi", path "C:/Users/XEnderMD/Desktop/CD Project Tools/Built/TimingDRV/Linux_x64/TimingDRV Engine.lvlib_Output Process/Main.vi", path "C:/Users/XEnderMD/Desktop/CD Project Tools/Built/TimingDRV/Linux_x64/TimingDRV Engine.lvlib_Output Process/Get Output Channel Values.vi", path "C:/Users/XEnderMD/Desktop/CD Project Tools/Built/TimingDRV/Linux_x64/TimingDRV Engine.lvlib_Sine Process/Get Output Channel Values.vi", path "C:/Users/XEnderMD/Desktop/CD Project Tools/Built/TimingDRV/Linux_x64/TimingDRV Engine.lvlib_Output Process/Set Output Channel Values.vi", path "C:/Users/XEnderMD/Desktop/CD Project Tools/Built/TimingDRV/Linux_x64/TimingDRV Engine.lvlib_Sine Process/Set Output Channel Values.vi", path "C:/Users/XEnderMD/Desktop/CD Project Tools/Built/TimingDRV/Linux_x64/TimingDRV Engine.lvlib_Output Process/Get Output FIFOs.vi", path "C:/Users/XEnderMD/Desktop/CD Project Tools/Built/TimingDRV/Linux_x64/TimingDRV Engine.lvlib_Sine Process/Get Output FIFOs.vi", path "C:/Users/XEnderMD/Desktop/CD Project Tools/Built/TimingDRV/Linux_x64/TimingDRV Engine.lvlib_Output Process/Set Output FIFOs.vi", path "C:/Users/XEnderMD/Desktop/CD Project Tools/Built/TimingDRV/Linux_x64/TimingDRV Engine.lvlib_Sine Process/Set Output FIFOs.vi", path "C:/Users/XEnderMD/Desktop/CD Project Tools/Built/TimingDRV/Linux_x64/TimingDRV Engine.lvlib_Sine Process/Configure.vi", path "C:/Users/XEnderMD/Desktop/CD Project Tools/Built/TimingDRV/Linux_x64/TimingDRV Engine.lvlib_Sine Process/Initialize.vi", path "C:/Users/XEnderMD/Desktop/CD Project Tools/Built/TimingDRV/Linux_x64/TimingDRV Engine.lvlib_Sine Process/Main.vi", path "C:/Users/XEnderMD/Desktop/CD Project Tools/Built/TimingDRV/Linux_x64/TimingDRV Engine.lvlib_Random Process/Get Output Channel Values.vi", path "C:/Users/XEnderMD/Desktop/CD Project Tools/Built/TimingDRV/Linux_x64/TimingDRV Engine.lvlib_Random Process/Set Output Channel Values.vi", path "C:/Users/XEnderMD/Desktop/CD Project Tools/Built/TimingDRV/Linux_x64/TimingDRV Engine.lvlib_Random Process/Get Output FIFOs.vi", path "C:/Users/XEnderMD/Desktop/CD Project Tools/Built/TimingDRV/Linux_x64/TimingDRV Engine.lvlib_Random Process/Set Output FIFOs.vi", path "C:/Users/XEnderMD/Desktop/CD Project Tools/Built/TimingDRV/Linux_x64/TimingDRV Engine.lvlib_Random Process/Configure.vi", path "C:/Users/XEnderMD/Desktop/CD Project Tools/Built/TimingDRV/Linux_x64/TimingDRV Engine.lvlib_Random Process/Initialize.vi", path "C:/Users/XEnderMD/Desktop/CD Project Tools/Built/TimingDRV/Linux_x64/TimingDRV Engine.lvlib_Random Process/Main.vi", path "C:/Users/XEnderMD/Desktop/CD Project Tools/Built/TimingDRV/Linux_x64/TimingDRV Engine.lvlib_Process/Configure.vi", path "C:/Users/XEnderMD/Desktop/CD Project Tools/Built/TimingDRV/Linux_x64/TimingDRV Engine.lvlib_Assembler/Launcher.vi", path "C:/Users/XEnderMD/Desktop/CD Project Tools/Built/TimingDRV/Linux_x64/TimingDRV Engine.lvlib_Process/Launcher.vi", path "C:/Users/XEnderMD/Desktop/CD Project Tools/Built/TimingDRV/Linux_x64/TimingDRV Engine.lvlib_Process/Initialize.vi", path "C:/Users/XEnderMD/Desktop/CD Project Tools/Built/TimingDRV/Linux_x64/TimingDRV Engine.lvlib_Process/Main.vi", path "C:/Users/XEnderMD/Desktop/CD Project Tools/Built/TimingDRV/Linux_x64/TimingDRV Engine.lvlib_Assembler/Shutdown.vi", path "C:/Users/XEnderMD/Desktop/CD Project Tools/Built/TimingDRV/Linux_x64/TimingDRV Engine.lvlib_Process/Shutdown.vi", path "C:/Users/XEnderMD/Desktop/CD Project Tools/Built/TimingDRV/Engine Release_depinstr.bin"]] ("Generated files 2"), "Project XML Editor in"=w4) -> ("error out"=w3:errorcluster, "Dependency Parameters"=w1:T1[], "Project XML Editor out"=w2:refnum<class "Project XML Editor.lvclass">)  [unwired: 6 in]
  "Array" <- w1
  n4 = for {
    shift-right: [w18] -> w10
    shift-left: w3 -> [w17]
    shift-right: [w19] -> w11
    shift-left: w2 -> [w16]
    tunnel: w1 -> [w15] mode=indexing
    n5 = call "Add XML Dependency.vi"("error in (no error)"=w17, "Dependency Parameters"=w15, "Project XML Editor in"=w16) -> ("error out"=w18:errorcluster, "Project XML Editor out"=w19:refnum<class "Project XML Editor.lvclass">)  [unwired: 7 in]
  }
  n6 = call "Destroy XML Editor.vi"("error in (no error)"=w10, "Project XML Editor in"=w11) -> ("error out"=→"error out":errorcluster)  [unwired: 9 in]
